vi "CAlex2_SetCuff_Shank_TreadmillLeft.vi"(9 "ExtraWeight":dbl, 10 "Distance To Knee":dbl=0.15, 11 "Shank Length":dbl=0.42 format="%#_13g") -> (3 "Shank Cuff":T1={"BodyID"=0, "CoM(CuffCS)"={"Coord4"=[0.0, 0.0, 0.0, 1.0], "ID"=0}, "Mass(kg)"=0.0, "CablePts(CuffCS)"=[], "Cuff->Body"=[[1.0, 0.0, 0.0, 0.0], [0.0, 1.0, 0.0, 0.0], [0.0, 0.0, 1.0, 0.0], [0.0, 0.0, 0.0, 1.0]]})   [LabVIEW 2016, in "CAlex2.lvclass"]
uses:
  CAlex2.lvclass
  SerialChain-Cable/TypeDef/Cuff.ctl
  SerialChain/TypeDef/PointOnBody.ctl
  <vilib>/Analysis/Matrix/Datatypes/RealMatrix.ctl
  SerialChain/TypeDef/xyzO.ctl
  <vilib>/Analysis/Matrix/NI_Matrix.lvlib
  SerialChain/SerialChain.lvclass
  SerialChain-Cable/SerialChain-Cable.lvclass
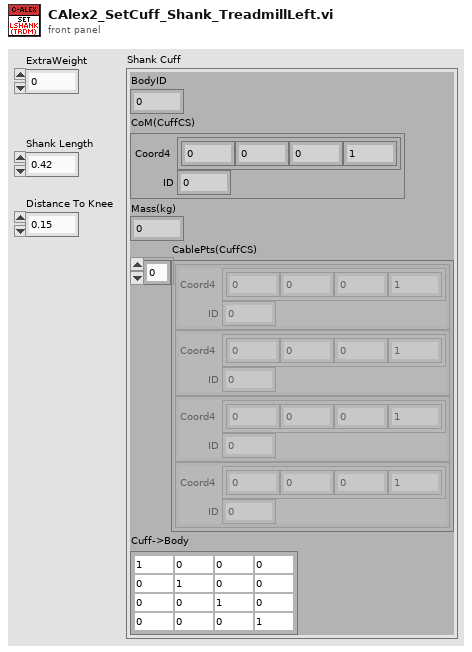
[diagram p1: front panel]
types:
  T1 = typedef "SerialChain-Cable.lvclass/Cuff.ctl" = cluster{"BodyID":i32, "CoM(CuffCS)":T2, "Mass(kg)":dbl, "CablePts(CuffCS)":T2[], "Cuff->Body":T3}
  T2 = typedef "SerialChain.lvclass/PointOnBody.ctl" = cluster{"Coord4":dbl[], "ID":i32}
  T3 = typedef "NI_Matrix.lvlib/RealMatrix.ctl" = dbl[][]
  T4 = typedef "SerialChain.lvclass/xyzO.ctl" = enum16{"X", "Y", "Z", "O"}
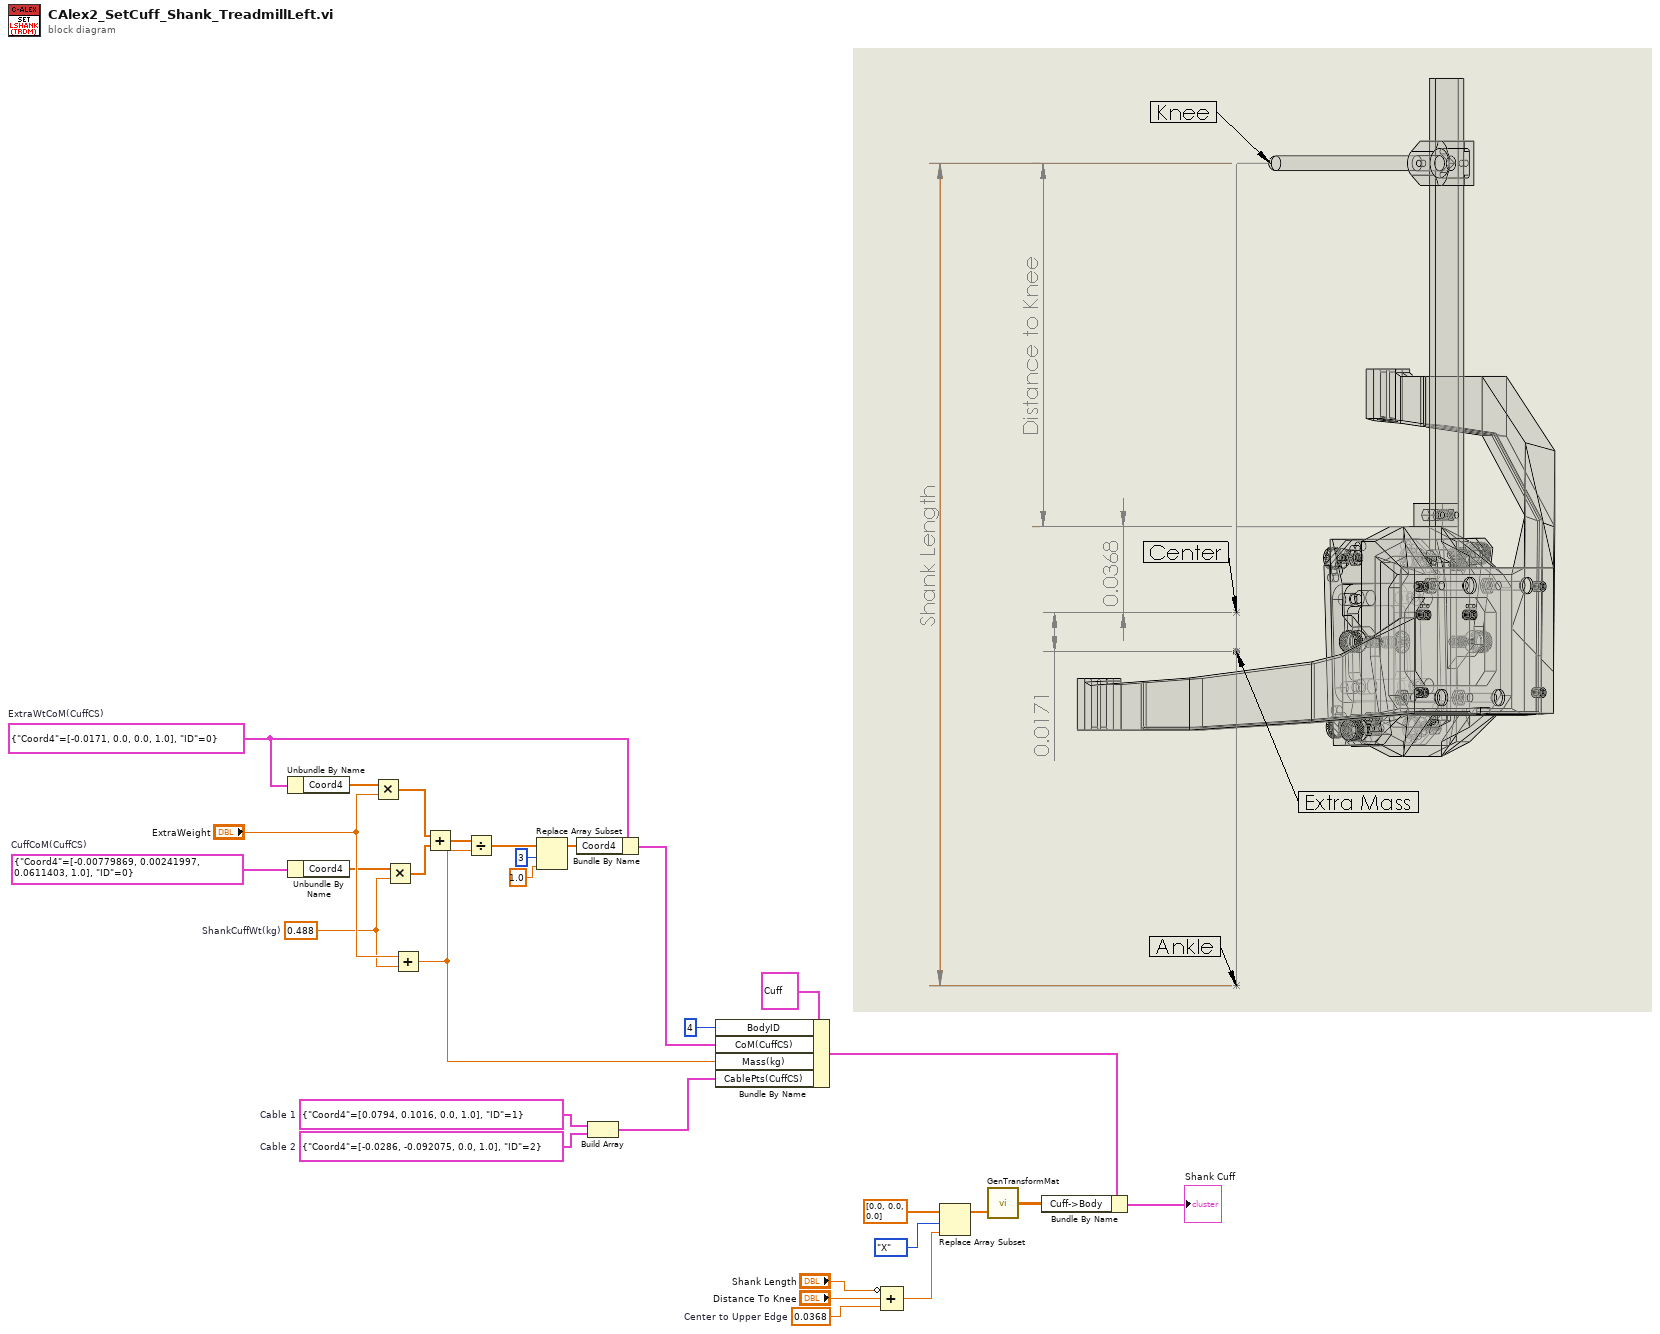
[diagram p0: block diagram]
diagram:
  w2 = 0.0368  # Center to Upper Edge
  w19 = T2 {"Coord4"=[-0.0171, 0.0, 0.0, 1.0], "ID"=0}  # ExtraWtCoM(CuffCS)
  w26 = T2 {"Coord4"=[-0.0286, -0.092075, 0.0, 1.0], "ID"=2}  # Cable 2
  w27 = T2 {"Coord4"=[0.0794, 0.1016, 0.0, 1.0], "ID"=1}  # Cable 1
  w11 = 0.488  # ShankCuffWt(kg)
  w13 = T2 {"Coord4"=[-0.00779869, 0.00241997, 0.0611403, 1.0], "ID"=0}  # CuffCoM(CuffCS)
  n1 = Unbundle By Name(w19) -> ("Coord4"=w25:dbl[])
  n2 = Unbundle By Name(w13) -> ("Coord4"=w23:dbl[])
  n3 = Multiply(x=w25, y="ExtraWeight") -> (x*y=w22:dbl[])
  n4 = Multiply(x=w23, y=w11) -> (x*y=w21:dbl[])
  n5 = Add(x="ExtraWeight", y=w11) -> (x+y=w12:dbl)
  n6 = Add(x=w22, y=w21) -> (x+y=w20:dbl[])
  n7 = Divide(x=w20, y=w12) -> (x/y=w18:dbl[])
  n8 = Replace Array Subset(array=w18, new element=1.0 ("new element/subarray"), index=3) -> (w17:dbl[])
  n9 = Bundle By Name(cluster=w19, "Coord4"=w17) -> (w14:T2)
  n10 = Build Array(w27, w26) -> (w28:T2[])
  n11 = Bundle By Name(cluster=T1 {"BodyID"=0, "CoM(CuffCS)"={"Coord4"=[0.0, 0.0, 0.0, 1.0], "ID"=0}, "Mass(kg)"=0.0, "CablePts(CuffCS)"=[], "Cuff->Body"=[[1.0, 0.0, 0.0, 0.0], [0.0, 1.0, 0.0, 0.0], [0.0, 0.0, 1.0, 0.0], [0.0, 0.0, 0.0, 1.0]]} ("Cuff Design"), "BodyID"=4, "CoM(CuffCS)"=w14, "Mass(kg)"=w12, "CablePts(CuffCS)"=w28) -> (w10:T1)
  n12 = Compound Arithmetic op=ADD(invert "Shank Length", "Distance To Knee", w2) -> (w1:dbl)
  n13 = Replace Array Subset(array=dbl[] [0.0, 0.0, 0.0], new element=w1, index=xyzO."X" ("XYZ")) -> (w7:dbl[])
  n14 = call "GenTransformMat.vi"("Translate 3Vector"=w7) -> ("Transformation Matrix"=w5:T3)  [unwired: 1 in]
  n15 = Bundle By Name(cluster=w10, "Cuff->Body"=w5) -> (→"Shank Cuff":T1)
